vi "train calculations test.vi"() -> ()   [LabVIEW 2009, in "Power Supply.lvclass"]
uses:
  Power Supply.lvclass
  Power Supply.lvclass/Power Supply.ctl
panel:
  in  "Train to Field":dbl[unit]=7.0
  in  "Original Field":dbl[unit]
  out "Rate Out":dbl[unit]=0.11666666666666667
  in  "Field":dbl[unit]
  in  "going up?":bool=TRUE
  out "Target Field":dbl[unit]
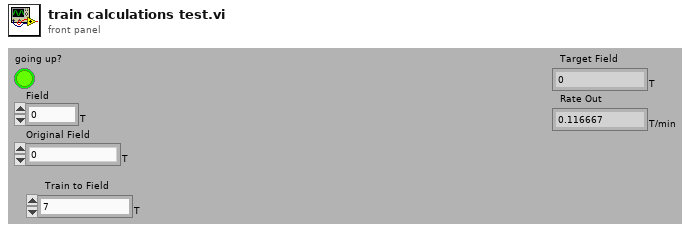
[diagram p1: front panel]
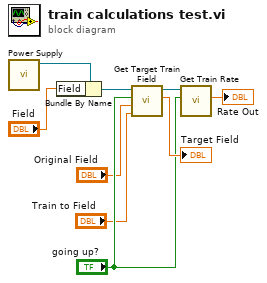
[diagram p0: block diagram]
diagram:
  n1 = call "Power Supply.vi"() -> ("Power Supply out"=w8:refnum<class "Power Supply.lvclass">)  [unwired: 10 in, 1 out]
  n2 = Bundle By Name(cluster=w8, "Field"="Field") -> (w3:refnum<class "Power Supply.lvclass">)
  n3 = call "Get Target Train Field.vi"("Train to Field"="Train to Field", "Original Field"="Original Field", "going up?"="going up?", "Power Supply in"=w3) -> ("Target Field"=→"Target Field":dbl[unit], "Power Supply Out"=w5:refnum<class "Power Supply.lvclass">)  [unwired: 6 in]
  n4 = call "Get Train Rate.vi"("going up?"="going up?", "Power Supply in"=w5) -> ("Rate Out"=→"Rate Out":dbl[unit])  [unwired: 8 in, 1 out]
